vi "Automated Tasks.vi"(0 "RB":bool, 2 "B":bool, 5 "Fire":bool, 7 "LB":bool, 9 "A":bool, 11 "Y":bool, 12 "X":bool, 13 "Back":bool) -> (3 "Fire":bool, 4 "Shooter":string, 6 "Winch":string, 10 "Case":string, 14 "Roller":string, 15 "Arm":string)   [LabVIEW 2013]
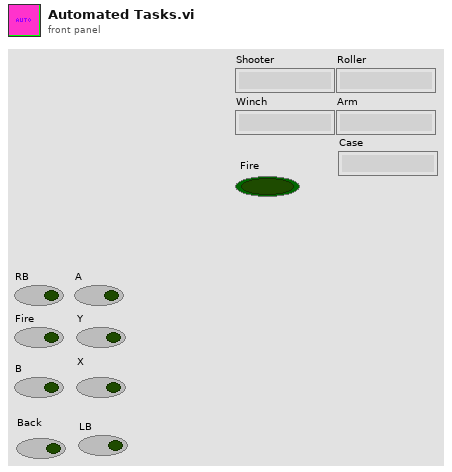
[diagram p1: front panel]
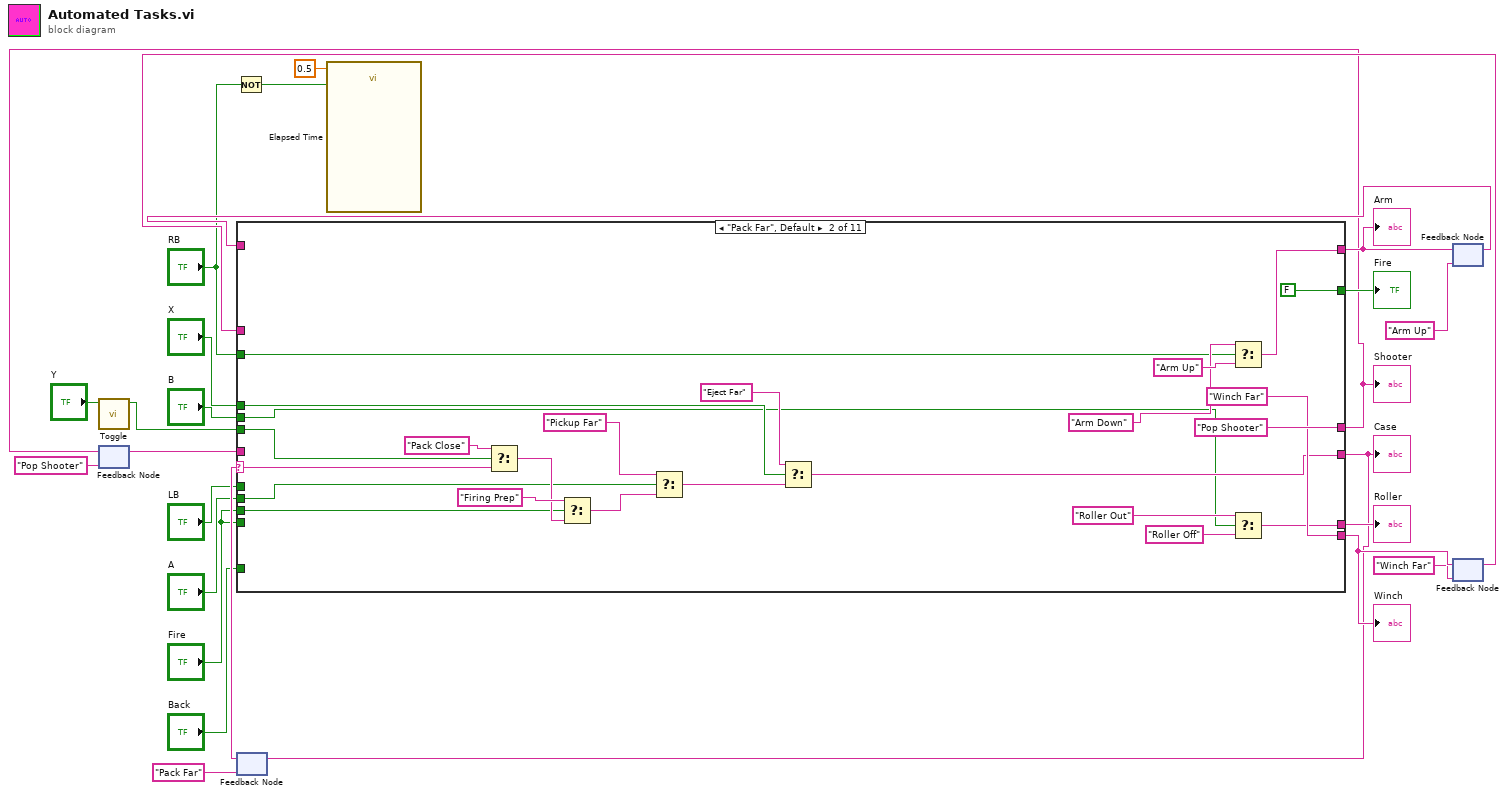
[diagram p0: block diagram]
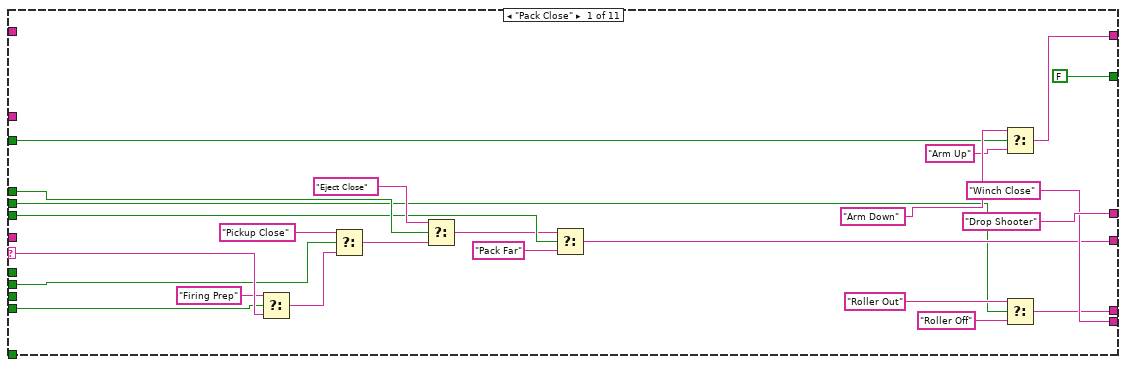
[diagram p2: hidden frame]
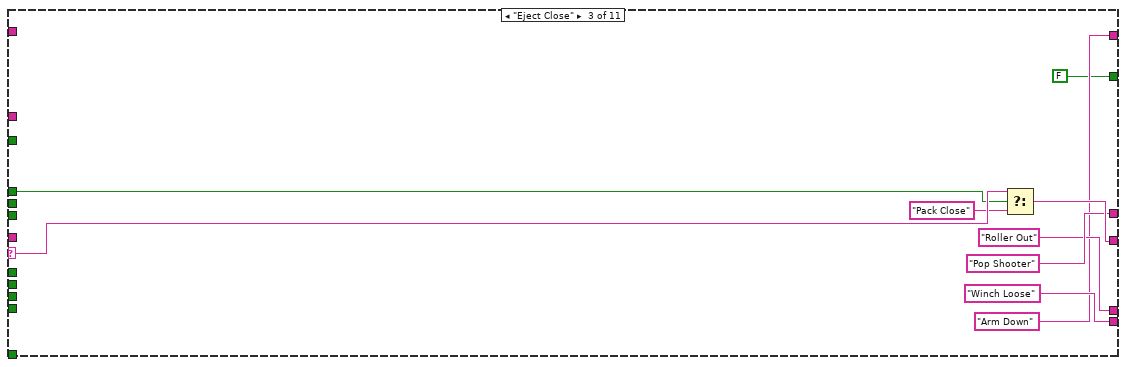
[diagram p3: hidden frame]
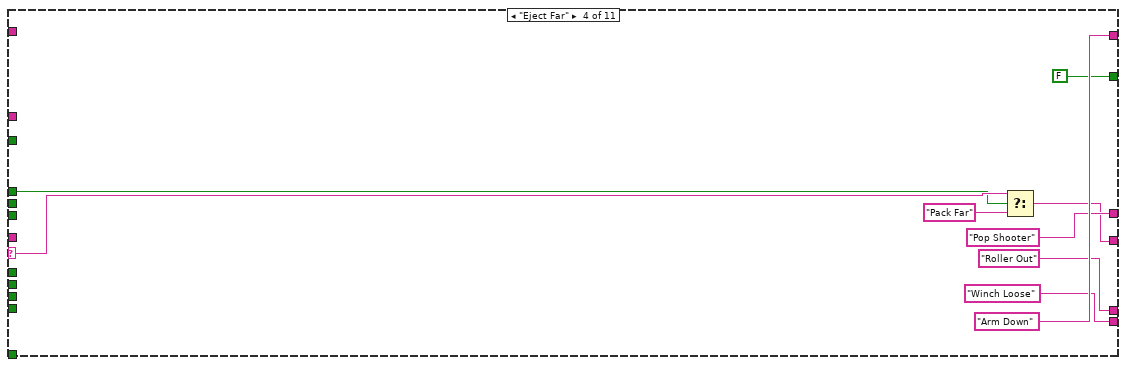
[diagram p4: hidden frame]
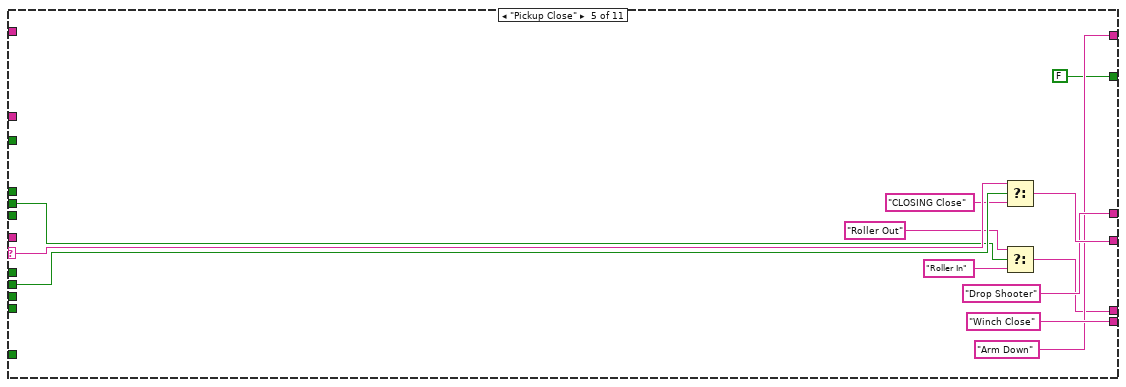
[diagram p5: hidden frame]
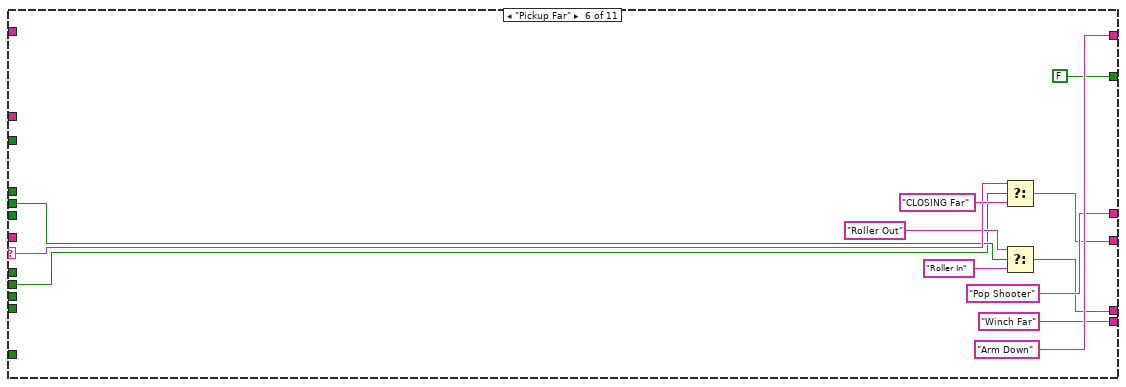
[diagram p6: hidden frame]
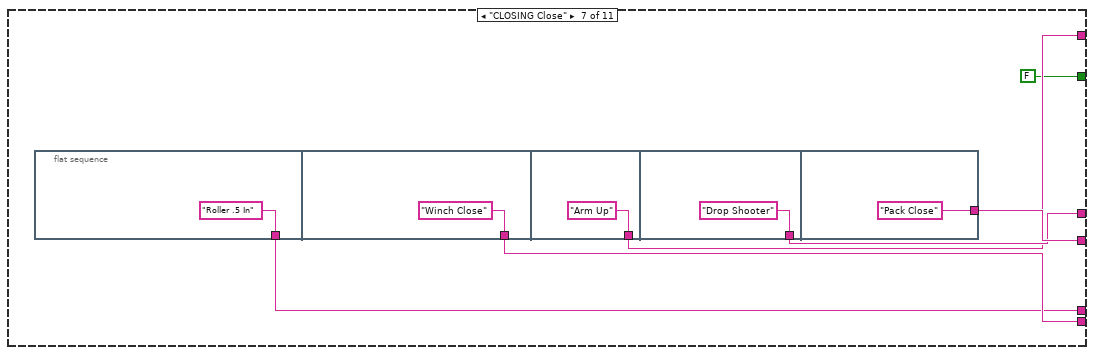
[diagram p7: hidden frame]
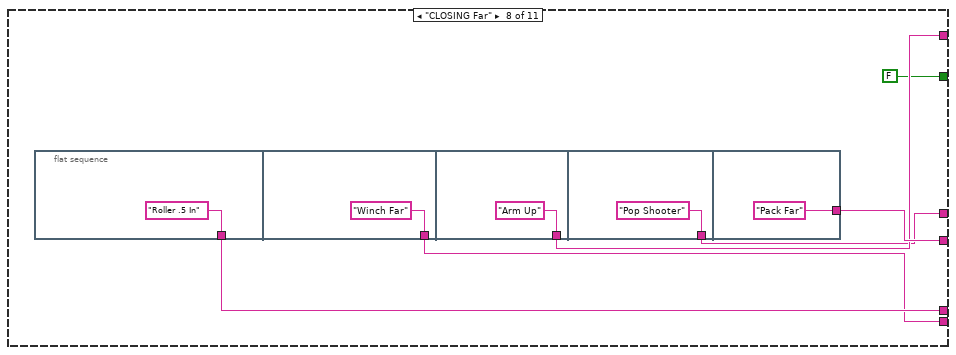
[diagram p8: hidden frame]
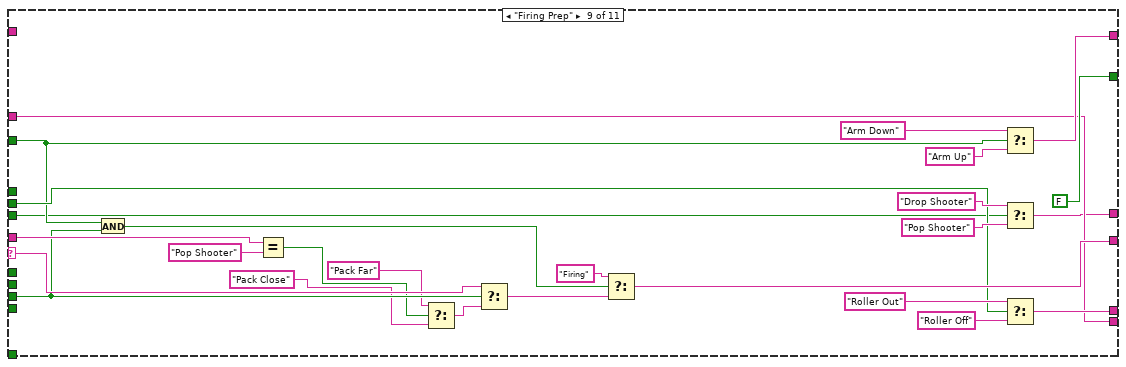
[diagram p9: hidden frame]
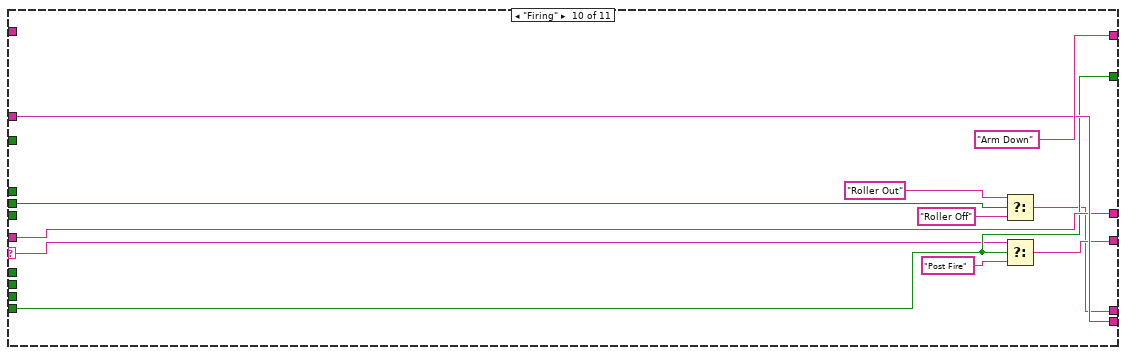
[diagram p10: hidden frame]
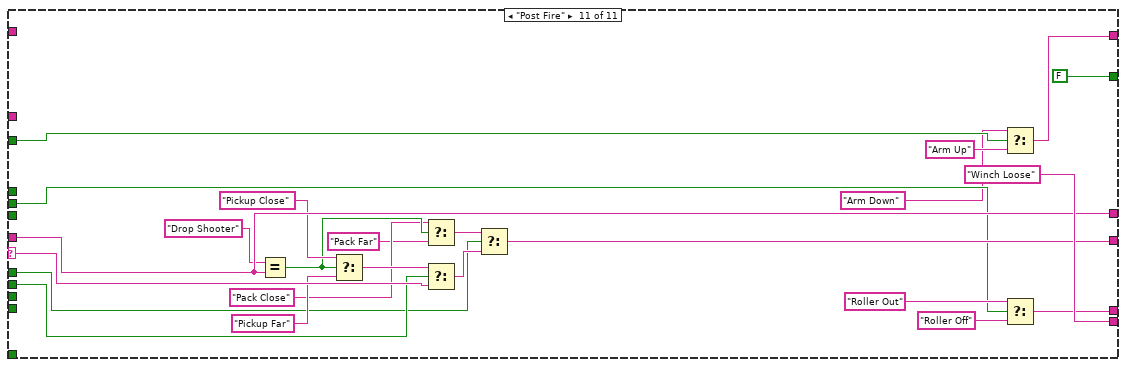
[diagram p11: hidden frame]
diagram:
  n1 = call "Toggle.vi"("Boolean"="Y") -> ("Toggled"=w1:bool)  [unwired: 10 in]
  n2 = feedback #1("Pop Shooter") -> (w19:string)
  n3 = Not(x="RB") -> (.not. x?=w8:bool)
  n4 = feedback #2("Pack Far" ("t")) -> (w25:string)
  n5 = call "Elapsed Time"("Time Target (s)"=0.5, "Reset"=w8) -> ()  [unwired: 10 in, 8 out]
  n6 = feedback #3("Arm Up") -> (w11:string)
  n7 = feedback #4("Winch Far") -> (w21:string)
  n8 = case shown="\"Pack Far\", Default" w25 {
    selector: w25 -> [w49 w51 w82 w85 w102 w110 _ _ w148 w169 w197]
    tunnel: "RB" -> [w36 w59 _ _ _ _ _ _ w146 _ w180]
    tunnel: [w39 w65 w80 w88 w100 w112 w121 w130 w159 w170 w186] -> w17
    tunnel: "A" -> [w46 w64 _ _ w103 w104 _ _ _ _ w176]
    tunnel: w1 -> [w28 w73 _ _ _ _ _ _ w139 _ _]
    tunnel: "B" -> [w30 w52 _ _ w94 w106 _ _ w152 w165 w182]
    tunnel: ["Drop Shooter" "Pop Shooter" "Pop Shooter" "Pop Shooter" "Drop Shooter" "Pop Shooter" w120 w128 w138 w172 w195] -> w6
    tunnel: ["Winch Close" "Winch Far" "Winch Loose" "Winch Loose" "Winch Close" "Winch Far" w118 w131 w150 w173 "Winch Loose"] -> w20
    tunnel: [w29 w53 "Roller Out" "Roller Out" w95 w107 w117 w132 w151 w164 w181] -> w22
    tunnel: [w42 w70 "Arm Down" "Arm Down" "Arm Down" "Arm Down" w119 w129 w161 "Arm Down" w178] -> w12
    tunnel: [FALSE FALSE FALSE FALSE FALSE FALSE FALSE FALSE FALSE w171 FALSE] -> w15
    tunnel: w21 -> [_ _ _ _ _ _ _ _ w150 w173 _]
    tunnel: w19 -> [_ _ _ _ _ _ _ _ w149 w172 w195]
    tunnel: "X" -> [w34 w57 w74 w83 _ _ _ _ _ _ _]
    tunnel: "Back" -> [_ _ _ _ _ _ _ _ _ _ _]
    tunnel: w11 -> [_ _ _ _ _ _ _ _ _ _ _]
    tunnel: "Fire" -> [_ w56 _ _ _ _ _ _ w145 _ _]
    tunnel: "Fire" -> [w33 _ _ _ _ _ _ _ _ w171 _]
    tunnel: "LB" -> [_ _ _ _ _ _ _ _ _ _ w175]
    frame "Pack Close" {
      n9 = Select(t="Firing Prep", s=w33, f=w49) -> (s? t:f=w47:string)
      n10 = Select(t="Pickup Close", s=w46, f=w47) -> (s? t:f=w44:string)
      n11 = Select(t="Eject Close", s=w34, f=w44) -> (s? t:f=w27:string)
      n12 = Select(t=w27, s=w28, f="Pack Far" ("t")) -> (s? t:f=w39:string)
      n13 = Select(t="Arm Down" ("f"), s=w36, f="Arm Up") -> (s? t:f=w42:string)
      n14 = Select(t="Roller Out", s=w30, f="Roller Off") -> (s? t:f=w29:string)
    }
    frame "Pack Far", Default {
      n15 = Select(t="Pack Close", s=w73, f=w51) -> (s? t:f=w68:string)
      n16 = Select(t="Firing Prep", s=w56, f=w68) -> (s? t:f=w66:string)
      n17 = Select(t="Pickup Far", s=w64, f=w66) -> (s? t:f=w67:string)
      n18 = Select(t="Eject Far", s=w57, f=w67) -> (s? t:f=w65:string)
      n19 = Select(t="Arm Down" ("f"), s=w59, f="Arm Up") -> (s? t:f=w70:string)
      n20 = Select(t="Roller Out", s=w52, f="Roller Off") -> (s? t:f=w53:string)
    }
    frame "Eject Close" {
      n21 = Select(t=w82, s=w74, f="Pack Close") -> (s? t:f=w80:string)
    }
    frame "Eject Far" {
      n22 = Select(t=w85, s=w83, f="Pack Far") -> (s? t:f=w88:string)
    }
    frame "Pickup Close" {
      n23 = Select(t=w102, s=w103, f="CLOSING Close") -> (s? t:f=w100:string)
      n24 = Select(t="Roller Out", s=w94, f="Roller In") -> (s? t:f=w95:string)
    }
    frame "Pickup Far" {
      n25 = Select(t=w110, s=w104, f="CLOSING Far") -> (s? t:f=w112:string)
      n26 = Select(t="Roller Out", s=w106, f="Roller In") -> (s? t:f=w107:string)
    }
    frame "CLOSING Close" {
      n27 = flat-sequence {
        tunnel: ["Roller .5 In"] -> w117
        tunnel: ["Winch Close"] -> w118
        tunnel: ["Arm Up"] -> w119
        tunnel: ["Drop Shooter"] -> w120
        tunnel: ["Pack Close"] -> w121
        frame #0 {
        }
        frame #1 {
        }
        frame #2 {
        }
        frame #3 {
        }
        frame #4 {
        }
      }
    }
    frame "CLOSING Far" {
      n28 = flat-sequence {
        tunnel: ["Roller .5 In"] -> w132
        tunnel: ["Winch Far"] -> w131
        tunnel: ["Arm Up"] -> w129
        tunnel: ["Pop Shooter"] -> w128
        tunnel: ["Pack Far"] -> w130
        frame #0 {
        }
        frame #1 {
        }
        frame #2 {
        }
        frame #3 {
        }
        frame #4 {
        }
      }
    }
    frame "Firing Prep" {
      n29 = And(x=w146, y=w145) -> (x .and. y?=w144:bool)
      n30 = Equal?(x=w149, y="Pop Shooter") -> (x = y?=w143:bool)
      n31 = Select(t="Pack Far" ("y"), s=w143, f="Pack Close" ("y")) -> (s? t:f=w142:string)
      n32 = Select(t=w148, s=w145, f=w142) -> (s? t:f=w147:string)
      n33 = Select(t="Firing", s=w144, f=w147) -> (s? t:f=w159:string)
      n34 = Select(t="Arm Down", s=w146, f="Arm Up" ("t")) -> (s? t:f=w161:string)
      n35 = Select(t="Drop Shooter" ("y"), s=w139, f="Pop Shooter") -> (s? t:f=w138:string)
      n36 = Select(t="Roller Out", s=w152, f="Roller Off") -> (s? t:f=w151:string)
    }
    frame "Firing" {
      n37 = Select(t="Roller Out", s=w165, f="Roller Off") -> (s? t:f=w164:string)
      n38 = Select(t=w169, s=w171, f="Post Fire") -> (s? t:f=w170:string)
    }
    frame "Post Fire" {
      n39 = Equal?(x="Drop Shooter", y=w195) -> (x = y?=w189:bool)
      n40 = Select(t="Pickup Close" ("x"), s=w189, f="Pickup Far" ("x")) -> (s? t:f=w196:string)
      n41 = Select(t="Pack Close" ("x"), s=w189, f="Pack Far" ("x")) -> (s? t:f=w190:string)
      n42 = Select(t=w196, s=w176, f=w197) -> (s? t:f=w191:string)
      n43 = Select(t=w190, s=w175, f=w191) -> (s? t:f=w186:string)
      n44 = Select(t="Arm Down" ("f"), s=w180, f="Arm Up") -> (s? t:f=w178:string)
      n45 = Select(t="Roller Out", s=w182, f="Roller Off") -> (s? t:f=w181:string)
    }
  }
  "Shooter" <- w6
  "Winch" <- w20
  "Roller" <- w22
  "Arm" <- w12
  "Case" <- w17
  "Fire" <- w15
  n46 = feedback-in #1(w6) -> ()
  n47 = feedback-in #2(w17) -> ()
  n48 = feedback-in #3(w12) -> ()
  n49 = feedback-in #4(w20) -> ()
